vi "open TCP Client.vi"(8 "error in (no error)":errorcluster caption="错误输入（无错误）", 11 "LS-H600-TCP Client 输入":refnum<class "LS-H600-TCP Client.lvclass">) -> (0 "error out":errorcluster caption="错误输出", 3 "LS-H600-TCP Client 输出":refnum<class "LS-H600-TCP Client.lvclass">)   [LabVIEW 2022 SP3, in "LS-H600-TCP Client.lvlib" / "LS-H600-TCP Client.lvclass"]
uses:
  LS-H600-TCP Client.lvclass
  C:/Program Files (x86)/National Instruments/LabVIEW 2022/vi.lib/ActorFramework/Actor/Actor.lvclass
  LS-H600-TCP Client.lvclass/LS-H600-TCP Client.ctl
  <vilib>/ActorFramework/Actor/Actor.lvclass/Actor.ctl
  <vilib>/ActorFramework/Message Enqueuer/Message Enqueuer.lvclass/Message Enqueuer.ctl
  <vilib>/ActorFramework/Message Enqueuer/Init from Existing Queue.vi
  <vilib>/ActorFramework/Message Enqueuer/Enqueue.vi
  C:/Program Files (x86)/National Instruments/LabVIEW 2022/vi.lib/ActorFramework/Message/Message.lvclass
  <vilib>/ActorFramework/Message Priority Queue/Priority Enqueue.vi
  <vilib>/ActorFramework/Message Enqueuer/Message Enqueuer.lvclass
  <vilib>/ActorFramework/Actor/Actor.lvclass
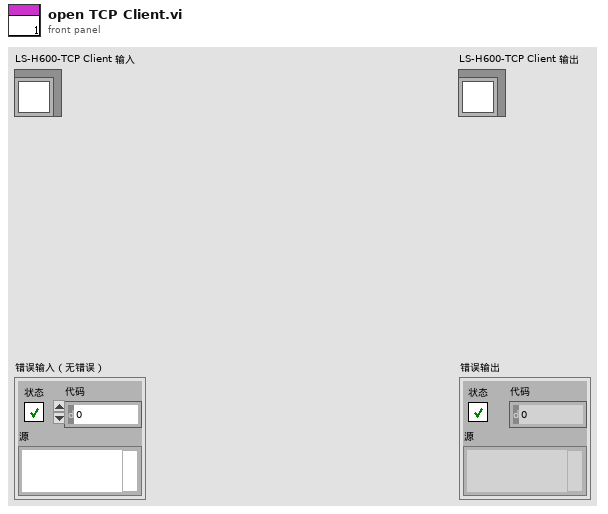
[diagram p1: front panel]
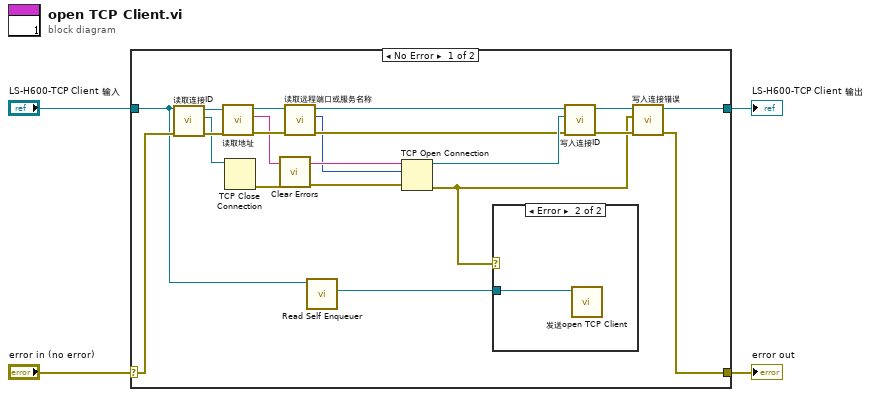
[diagram p0: block diagram]
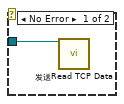
[diagram p2: hidden frame]
diagram:
  n1 = case shown="No Error" "error in (no error)" {
    selector: "error in (no error)" -> [w12 w28]
    tunnel: [w16 w28] -> w3
    tunnel: [w17 w27] -> w1
    tunnel: "LS-H600-TCP Client 输入" -> [w6 w27]
    frame No Error {
      n2 = call "读取连接ID.vi"("error in (no error)"=w12, "LS-H600-TCP Client输入"=w6) -> ("error out"=w11:errorcluster, "连接ID"=w10:refnum<k5>, "LS-H600-TCP Client输出"=w13:refnum<class "LS-H600-TCP Client.lvclass">)  [unwired: 7 in]
      n3 = call "读取地址.vi"("error in (no error)"=w11, "LS-H600-TCP Client输入"=w13) -> ("error out"=w21:errorcluster, "地址"=w15:string, "LS-H600-TCP Client输出"=w24:refnum<class "LS-H600-TCP Client.lvclass">)  [unwired: 7 in]
      n4 = TCP Close Connection(connection ID=w10) -> (error out=w9:errorcluster)  [unwired: 2 in, 1 out]
      n5 = call <vilib>:"Clear Errors.vi"("error in (no error)"=w9) -> ("error out"=w8:errorcluster)  [unwired: 5 in, 1 out]
      n6 = call "读取远程端口或服务名称.vi"("error in (no error)"=w21, "LS-H600-TCP Client输入"=w24) -> ("error out"=w20:errorcluster, "远程端口或服务名称"=w14:u16, "LS-H600-TCP Client输出"=w23:refnum<class "LS-H600-TCP Client.lvclass">)  [unwired: 7 in]
      n7 = call <vilib>:"Read Self Enqueuer.vi"("Actor"=w6) -> ("Self Enqueuer"=w5:refnum<class "Message Enqueuer.lvclass">)  [unwired: 10 in]
      n8 = TCP Open Connection(address=w15, remote port or service name=w14, error in (no error)=w8) -> (connection ID=w22:refnum<k5>, error out=w7:errorcluster)  [unwired: 2 in]
      n9 = case shown="Error" w7 {
        tunnel: w5 -> [w25 w26]
        frame No Error {
          n10 = call "发送Read TCP Data.vi"("Message Enqueuer"=w25) -> ()  [unwired: 9 in, 2 out]
        }
        frame Error {
          n11 = call "发送open TCP Client.vi"("Message Enqueuer"=w26) -> ()  [unwired: 9 in, 2 out]
        }
      }
      n12 = call "写入连接ID.vi"("error in (no error)"=w20, "连接ID"=w22, "LS-H600-TCP Client输入"=w23) -> ("error out"=w18:errorcluster, "LS-H600-TCP Client输出"=w19:refnum<class "LS-H600-TCP Client.lvclass">)  [unwired: 7 in]
      n13 = call "写入连接错误.vi"("error in (no error)"=w18, "连接错误"=w7, "LS-H600-TCP Client输入"=w19) -> ("error out"=w16:errorcluster, "LS-H600-TCP Client输出"=w17:refnum<class "LS-H600-TCP Client.lvclass">)  [unwired: 7 in]
    }
    frame Error {
    }
  }
  "error out" <- w3
  "LS-H600-TCP Client 输出" <- w1
